vi "PLC.WaitForConfirm.vi"(8 "error in":errorcluster, 11 "Data_in":T1={"Status"={"Idx"=0, "ConnRef"=0, "State"=enum."Off", "LiveBitTimer"=timestamp(0 s since 1904-01-01)}, "Sets"={"Enable"=FALSE, "IP"="", "Rack"=0, "Slot"=0, "LifeBitTimer_s"=0.0, "DataBlockAddr_PCStatus"=0, "DataBlockAddr_PLCStatus"=1, "DataBlockAddr_PLCNewData"=[], "DataBlockSize_PLCNewData"=[], "DataBlockAddr_PLCChangeOver"=[], "DataBlockSize_PLCChangeOver"=[], "DataBlockAddr_PCChangeOver"=[], "DataBlockAddr_PLCCheckStatus"=[], "DataBlockSize_PLCCheckStatus"=[], "DataBlockAddr_PCCheckStatus"=[]}, "PCstatus"={"General"={"LifeBit"=FALSE, "DbRun"=FALSE}, "Stations"=[]}, "PLCstatus"={"General"={"LifeBit"=FALSE}, "Stations"=[]}}) -> (0 "error out":errorcluster, 2 "Confirmed?":bool, 3 "Data_out":T1={"Status"={"Idx"=0, "ConnRef"=0, "State"=enum."Off", "LiveBitTimer"=timestamp(0 s since 1904-01-01)}, "Sets"={"Enable"=FALSE, "IP"="", "Rack"=0, "Slot"=0, "LifeBitTimer_s"=0.0, "DataBlockAddr_PCStatus"=0, "DataBlockAddr_PLCStatus"=1, "DataBlockAddr_PLCNewData"=[], "DataBlockSize_PLCNewData"=[], "DataBlockAddr_PLCChangeOver"=[], "DataBlockSize_PLCChangeOver"=[], "DataBlockAddr_PCChangeOver"=[], "DataBlockAddr_PLCCheckStatus"=[], "DataBlockSize_PLCCheckStatus"=[], "DataBlockAddr_PCCheckStatus"=[]}, "PCstatus"={"General"={"LifeBit"=FALSE, "DbRun"=FALSE}, "Stations"=[]}, "PLCstatus"={"General"={"LifeBit"=FALSE}, "Stations"=[]}})   [LabVIEW 2016]
doc: "Read data block from PLC to PC and write data block from PC to PLC. Control live bit of PC\n\nWabco 2017 All right reserved\nAuthor: maciej.szupienko@wabco-auto.com"
uses:
  PLC.Data.ctl
  PLC.Data.Status.ctl
  PLC.State.ctl
  PLC.Data.Sets.ctl
  LowLevel/PLC.DataBlock.PCstatus.ctl
  LowLevel/PLC.DataBlock.PCstatus.General.ctl
  LowLevel/PLC.DataBlock.PCstatus.Station.ctl
  LowLevel/PLC.DataBlock.PLCstatus.ctl
  LowLevel/PLC.DataBlock.PLCstatus.General.ctl
  LowLevel/PLC.DataBlock.PLCstatus.Station.ctl
  Tools/EventLog/EventLog.EventSource.ctl
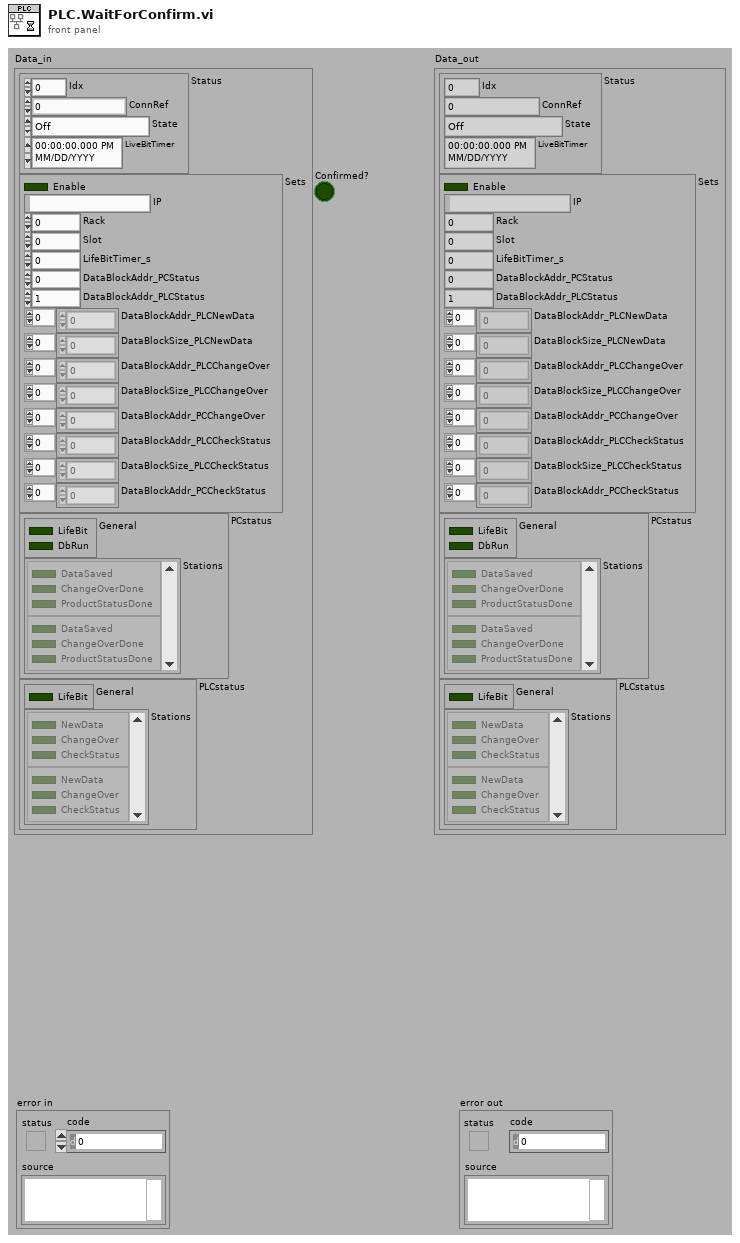
[diagram p1: front panel]
types:
  T1 = typedef "PLC.Data.ctl" = cluster{"Status":T2, "Sets":T4, "PCstatus":T5, "PLCstatus":T8}
  T2 = typedef "PLC.Data.Status.ctl" = cluster{"Idx":i32, "ConnRef":u64, "State":T3, "LiveBitTimer":timestamp}
  T3 = typedef "PLC.State.ctl" = enum32{"Off", "Error", "Idle", "Run"}
  T4 = typedef "PLC.Data.Sets.ctl" = cluster{"Enable":bool, "IP":string, "Rack":i32, "Slot":i32, "LifeBitTimer_s":dbl, "DataBlockAddr_PCStatus":i32, "DataBlockAddr_PLCStatus":i32, "DataBlockAddr_PLCNewData":i32[], "DataBlockSize_PLCNewData":i32[], "DataBlockAddr_PLCChangeOver":i32[], "DataBlockSize_PLCChangeOver":i32[], "DataBlockAddr_PCChangeOver":i32[], "DataBlockAddr_PLCCheckStatus":i32[], "DataBlockSize_PLCCheckStatus":i32[], "DataBlockAddr_PCCheckStatus":i32[]}
  T5 = typedef "PLC.DataBlock.PCstatus.ctl" = cluster{"General":T6, "Stations":T7[]}
  T6 = typedef "PLC.DataBlock.PCstatus.General.ctl" = cluster{"LifeBit":bool, "DbRun":bool}
  T7 = typedef "PLC.DataBlock.PCstatus.Station.ctl" = cluster{"DataSaved":bool, "ChangeOverDone":bool, "ProductStatusDone":bool}
  T8 = typedef "PLC.DataBlock.PLCstatus.ctl" = cluster{"General":T9, "Stations":T10[]}
  T9 = typedef "PLC.DataBlock.PLCstatus.General.ctl" = cluster{"LifeBit":bool}
  T10 = typedef "PLC.DataBlock.PLCstatus.Station.ctl" = cluster{"NewData":bool, "ChangeOver":bool, "CheckStatus":bool}
  T11 = typedef "EventLog.EventSource.ctl" = enum16{"All", "Gui", "Cache", "PLC1", "PLC2", "PLC3", "DB", "DB01", "DB02", "DB03", "DB04", "DB05", "DB06", "DB07", "DB08", "DB09", "DB10", "DB11", "DB12", "DB13", "DB14", "DB15", "DB16"}
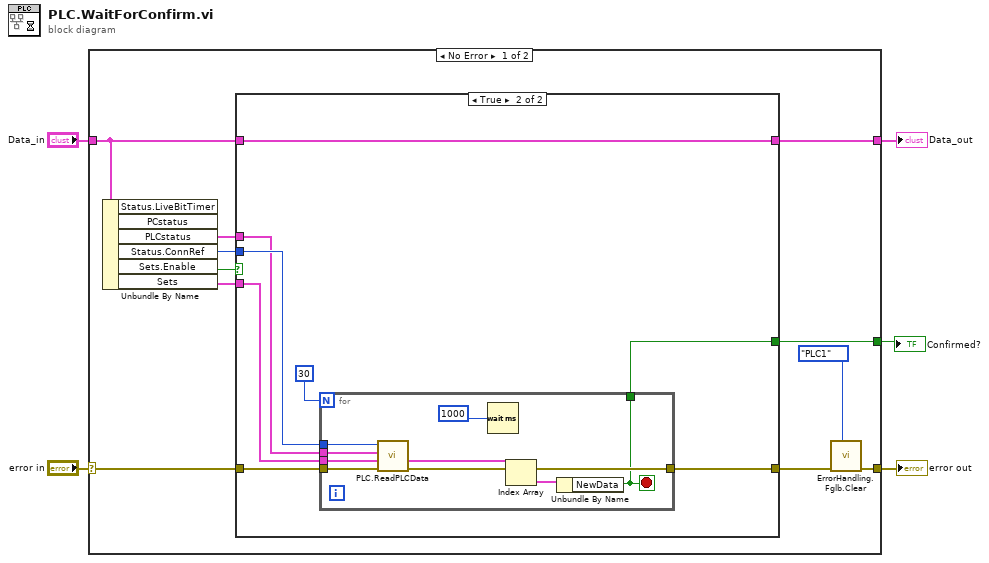
[diagram p0: block diagram]
diagram:
  n1 = case shown="No Error" "error in" {
    selector: "error in" -> [w13 w37]
    tunnel: [w15 w37] -> w2
    tunnel: "Data_in" -> [w14 w36]
    tunnel: [w16 w36] -> w4
    tunnel: [w6 _] -> w1
    frame No Error {
      n2 = Unbundle By Name(w14) -> ("PLCstatus"=w10:T8, "Status.ConnRef"=w12:u64, "Sets.Enable"=w9:bool, "Sets"=w8:T4)  [unwired: 2 out]
      n3 = case shown="True" w9 {
        tunnel: [w18 w22] -> w16
        tunnel: w14 -> [w18 w22]
        tunnel: w13 -> [w17 w24]
        tunnel: w12 -> [_ w26]
        tunnel: [w17 w21] -> w11
        tunnel: w10 -> [_ w25]
        tunnel: w8 -> [_ w23]
        tunnel: [_ w19] -> w6
        frame False {
        }
        frame True {
          n4 = for {
            N: 30 -> [_]
            tunnel: w26 -> [w35]
            tunnel: w25 -> [w34]
            tunnel: w24 -> [w33]
            tunnel: w23 -> [w32]
            tunnel: [w29] -> w21
            tunnel: [w27] -> w19
            stop <- w27 stop-if-true
            n5 = call "PLC.ReadPLCData.vi"("error in (no error)"=w33, "Sets"=w32, "PLCdata in"=w34, "Ref in"=w35) -> ("error out"=w29:errorcluster, "Events"=w31:T10[])  [unwired: 4 in, 2 out]
            n6 = Wait (ms)(milliseconds to wait=1000) -> ()  [unwired: 1 out]
            n7 = Index Array(array=w31) -> (element=w30:T10)  [unwired: 1 in]
            n8 = Unbundle By Name(w30) -> ("NewData"=w27:bool)
          }
        }
      }
      n9 = call "ErrorHandling.Fglb.Clear.vi"("Event source"=EventLog.EventSource."PLC1", "error in (no error)"=w11) -> ("error out"=w15:errorcluster)  [unwired: 9 in]
    }
    frame Error {
    }
  }
  "error out" <- w2
  "Data_out" <- w4
  "Confirmed?" <- w1
